vi "一维数组排序返回索引.vi"(8 "error in (no error)":errorcluster caption="错误输入（无错误）", 11 "输入":dbl[](array[numeric])) -> (0 "error out":errorcluster caption="错误输出", 2 "排序索引":i32[](array[numeric]), 3 "输出":dbl[](array[numeric]))   [LabVIEW 2014]
doc: "该模板用于创建子VI。"
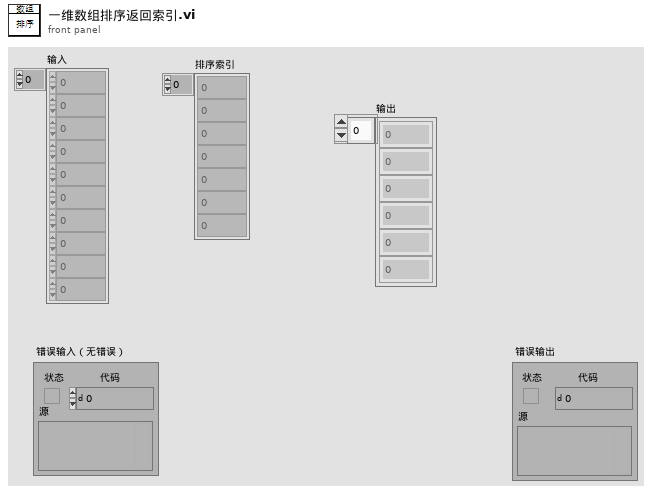
[diagram p1: front panel]
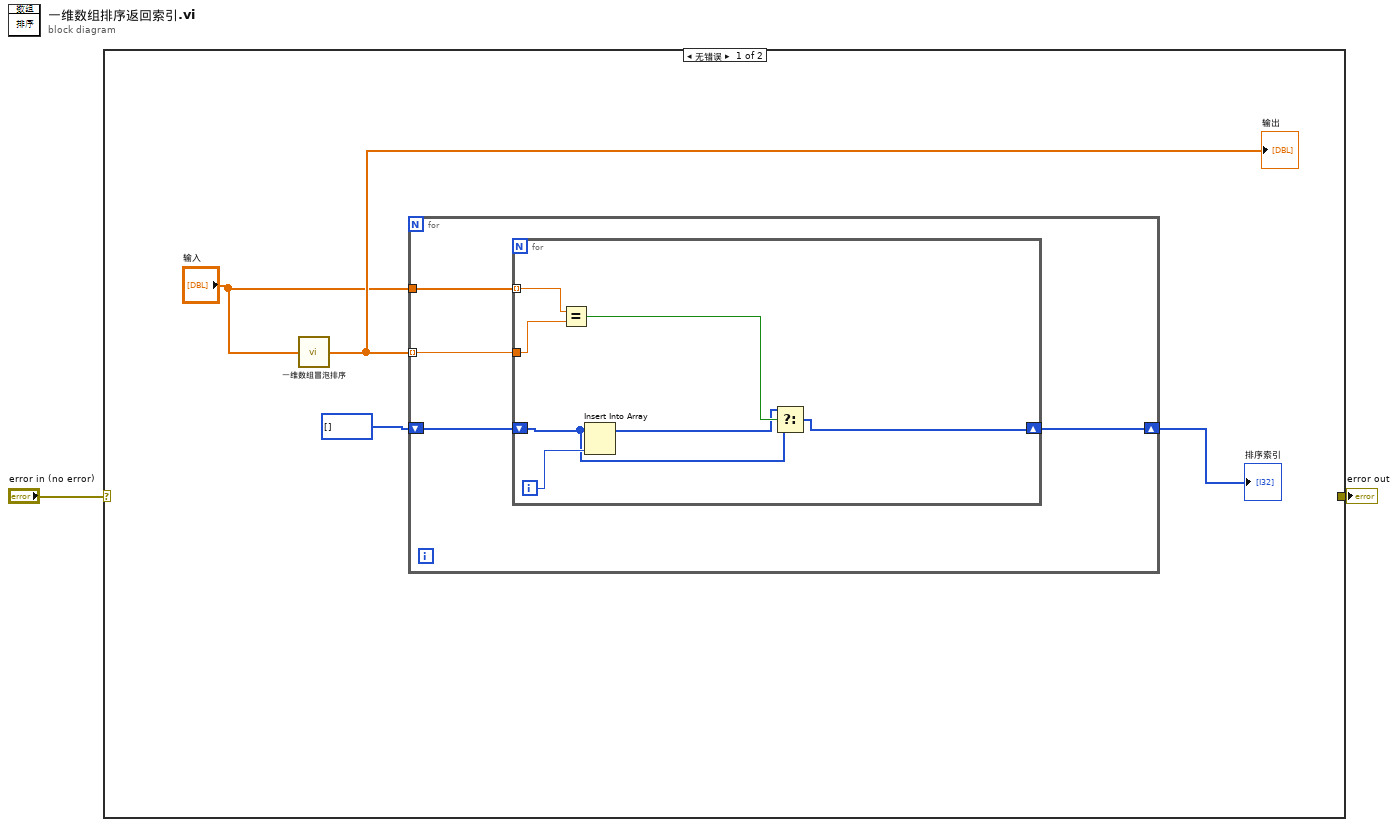
[diagram p0: block diagram]
diagram:
  n1 = case shown="无错误" "error in (no error)" {
    selector: "error in (no error)" -> [_ w18]
    tunnel: [_ w18] -> w1
    frame No Error {
      n2 = call "一维数组冒泡排序.vi"("输入"="输入") -> ("输出"=w6:dbl[])
      "输出" <- w6
      n3 = for {
        tunnel: w6 -> [w9] mode=indexing
        tunnel: "输入" -> [w10]
        shift-right: [w7] -> w3
        shift-left: i32[] [] -> [w8]
        n4 = for {
          tunnel: w10 -> [w17] mode=indexing
          tunnel: w9 -> [w16]
          shift-right: [w11] -> w7
          shift-left: w8 -> [w12]
          i -> [w14]
          n5 = Equal?(x=w17, y=w16) -> (x = y?=w15:bool)
          n6 = Insert Into Array(array=w12, new element=w14) -> (w13:i32[])  [unwired: 1 in]
          n7 = Select(t=w13, s=w15, f=w12) -> (s? t:f=w11:i32[])
        }
      }
      "排序索引" <- w3
    }
    frame Error {
    }
  }
  "error out" <- w1
